vi "Mem_StrArray.vi"(8 "error in (no error)":errorcluster, 11 "dataInfo":T1) -> (0 "error out":errorcluster, 2 "SreArray":string[](array[string]))   [LabVIEW 2019, in "Memory Data Access.lvlib"]
uses:
  Memory Data Access.lvlib
  Typedef/memoryDataBlock.ctl
  Global/Global.vi
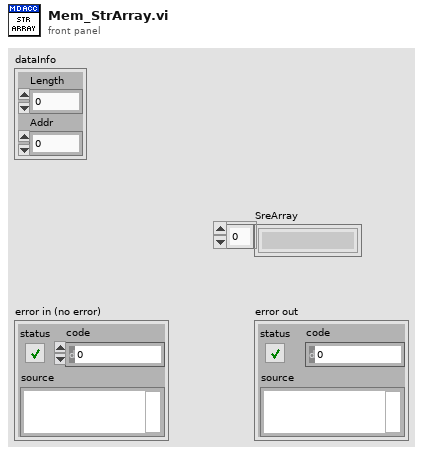
[diagram p1: front panel]
types:
  T1 = typedef "Memory Data Access.lvlib/memoryDataBlock.ctl" = cluster{"Length":u32, "Addr":u64}
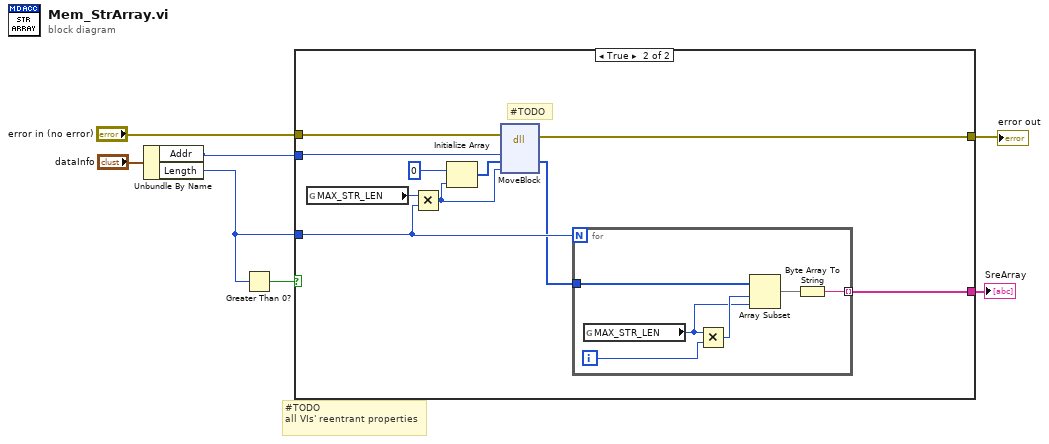
[diagram p0: block diagram]
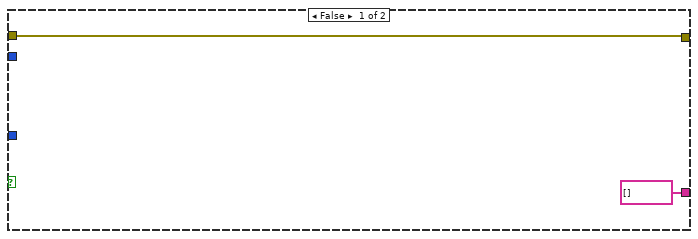
[diagram p2: hidden frame]
diagram:
  # "#TODO\nall VIs' reentrant properties"
  n1 = Unbundle By Name("dataInfo") -> ("Addr"=w3:u64, "Length"=w2:u32)
  n2 = Greater Than 0?(x=w2) -> (x > 0?=w5:bool)
  n3 = case shown="True" w5 {
    tunnel: "error in (no error)" -> [w9 w19]
    tunnel: [w9 w11] -> w6
    tunnel: w3 -> [_ w17]
    tunnel: w2 -> [_ w14]
    tunnel: [string[] [] w12] -> w1
    frame False {
    }
    frame True {
      # "#TODO"
      n4 = global read "Global.vi" "MAX_STR_LEN"() -> (w15:u32)
      n5 = Multiply(x=w15, y=w14) -> (x*y=w10:u32)
      n6 = Initialize Array(u8 0, w10) -> (w18:u8[])
      n7 = dll-call lib="LabVIEW" fn="MoveBlock"(error in=w19, "Address"=w17, "Destination"=w18, "Size"=w10) -> (error out=w11:errorcluster, "Destination"=w13:u8[])  [unwired: 5 in, 1 out]
      n8 = for {
        N: w14 -> [_]
        tunnel: w13 -> [w25]
        tunnel: [w20] -> w12 mode=indexing
        i -> [w24]
        n9 = global read "Global.vi" "MAX_STR_LEN"() -> (w22:u32)
        n10 = Multiply(x=w22, y=w24) -> (x*y=w23:u32)
        n11 = Array Subset(array=w25, index=w23, length=w22) -> (w21:u8[])
        n12 = Byte Array To String(unsigned byte array=w21) -> (string=w20:string)
      }
    }
  }
  "error out" <- w6
  "SreArray" <- w1
